vi "testEvaluate.vi"() -> ()   [LabVIEW 2019, in "ConstraintTest.lvlib" / "Constraint.lvlib"]
uses:
  Constraint.lvlib
  Constraint/Constraint/Constraint.lvclass
  Assertion/Assertion.lvlib
panel:
  out "error out":errorcluster
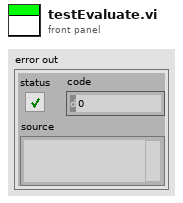
[diagram p1: front panel]
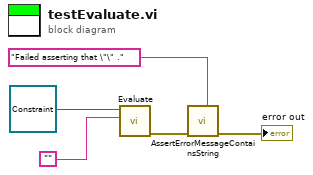
[diagram p0: block diagram]
diagram:
  n1 = call-dynamic "Evaluate.vi"("Actual"="", "Constraint in"=refnum<class "Constraint.lvclass"> refnum ("Constraint.lvlib:Constraint.lvclass")) -> ("error out"=w3:errorcluster)  [unwired: 8 in, 1 out]
  n2 = call "AssertErrorMessageContainsString.vi"("Expected"="Failed asserting that \"\" .", "error in (no error)"=w3) -> ("error out"=→"error out":errorcluster)  [unwired: 9 in]
